vi "Shoulder Position to Target Wrist Angle.vi"(7 "Shoulder Max Enc":dbl, 8 "Wanted Wrist Angle (-1, 1)":dbl(knob) scale=1.0..-1.0, 9 "Shoulder Enc Positon":dbl(slide) scale=0.0..360000.0, 11 "Shoulder Min Enc":dbl) -> (1 "Target Wrist Angle deg(90-270)":dbl(knob) scale=0.0..360.0)   [LabVIEW 2023]
panel:
  out "Numeric 2":dbl
  out "Numeric":dbl
  out "Shoulder Angle":dbl(knob)
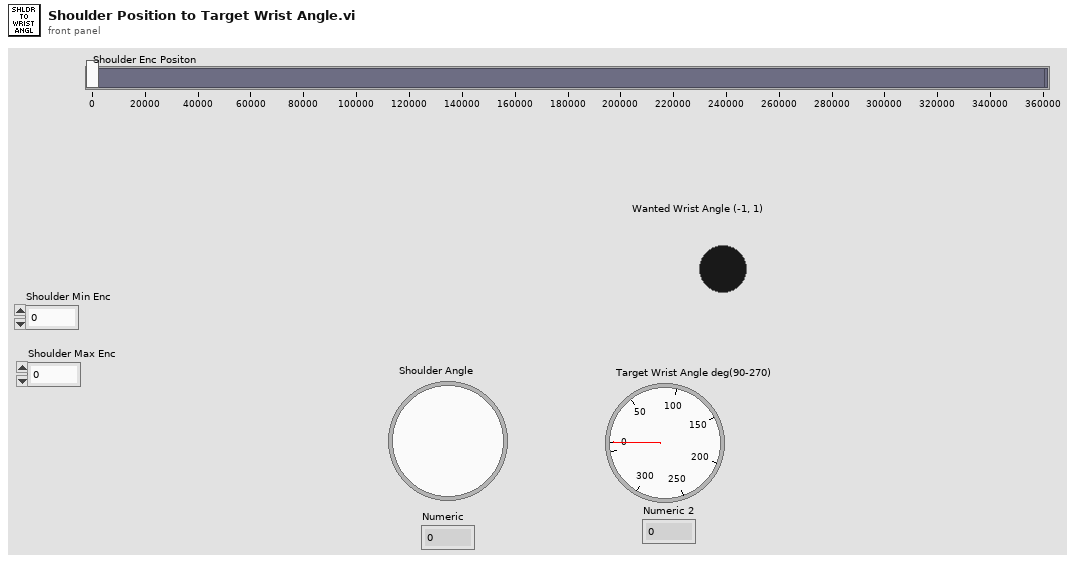
[diagram p1: front panel]
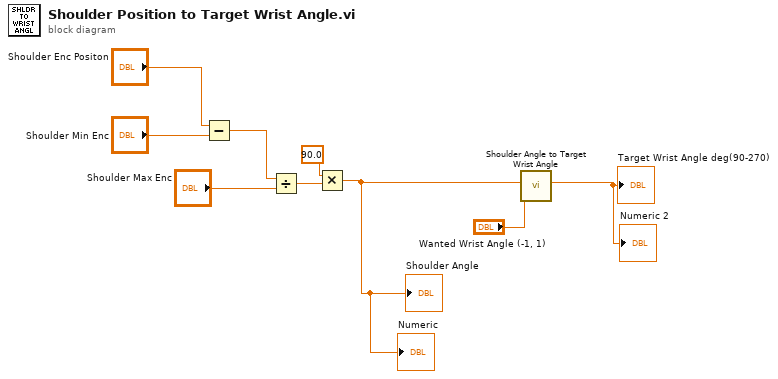
[diagram p0: block diagram]
diagram:
  n1 = Subtract(x="Shoulder Enc Positon", y="Shoulder Min Enc") -> (x-y=w7:dbl)
  n2 = Divide(x=w7, y="Shoulder Max Enc") -> (x/y=w5:dbl)
  n3 = Multiply(x=90.0, y=w5) -> (x*y=w3:dbl)
  "Shoulder Angle" <- w3
  "Numeric" <- w3
  n4 = call "Shoulder Angle to Target Wrist Angle.vi"("Target Wrist Angle (-1,1)"="Wanted Wrist Angle (-1, 1)", "Shoulder angle deg(0-180)"=w3) -> ("Target Wrist angle deg(90-270)"=→"Numeric 2" →"Target Wrist Angle deg(90-270)":dbl)  [unwired: 9 in]
